vi "ControlPanel(noobjects.vi"() -> ()   [LabVIEW 2017]
panel:
  out "boot up output":string="\r\n"
  in  "Read":bool
  in  "Inhibit":bool
  in  "Change Wavelength in nm":bool
  in  "Change Retardance in nm":bool
  in  "Change Retardance in wave units":bool
  in  "Input":dbl
  out "Wavelength":dbl[unit]
  out "Retardation in nm":dbl[unit]
  out "Retardation in wave units":dbl
  in  "stop":bool
  out "error out":errorcluster
  in  "error in (no error)":errorcluster
  in  "Factory Reset":bool
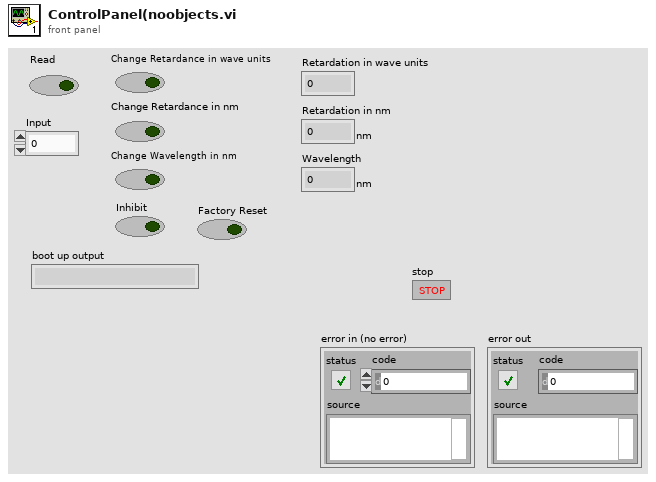
[diagram p1: front panel]
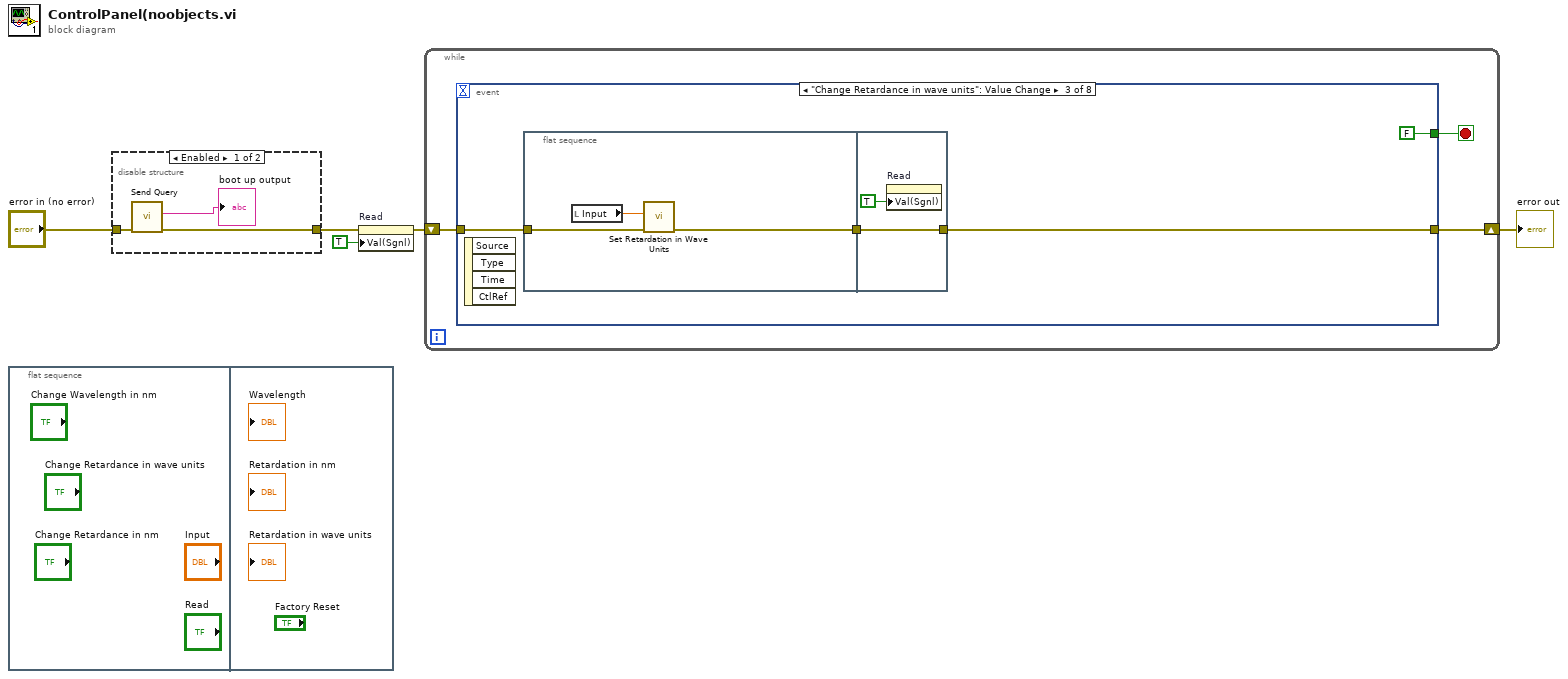
[diagram p0: block diagram]
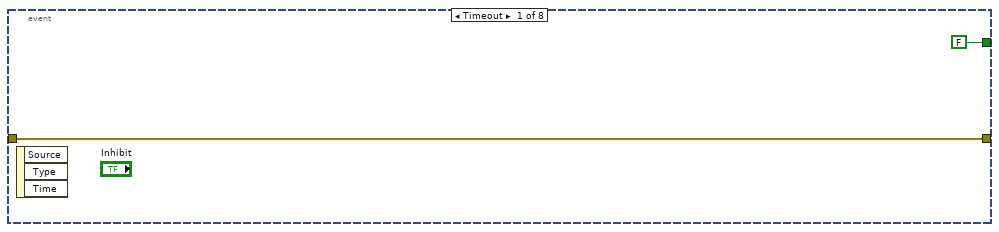
[diagram p3: hidden frame]
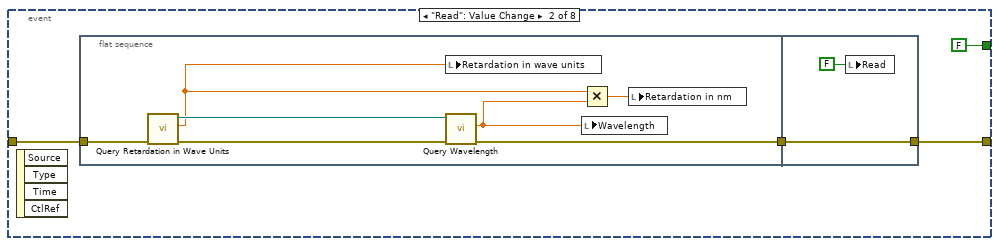
[diagram p4: hidden frame]
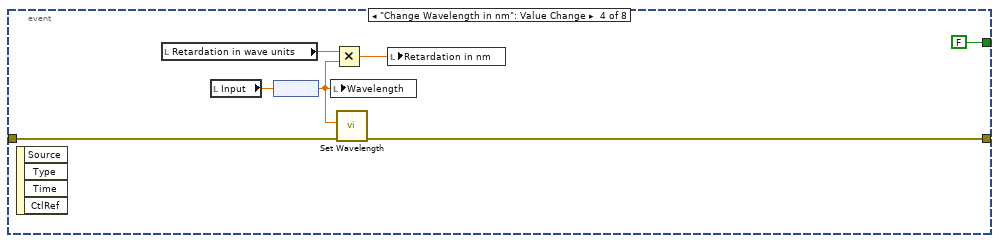
[diagram p5: hidden frame]
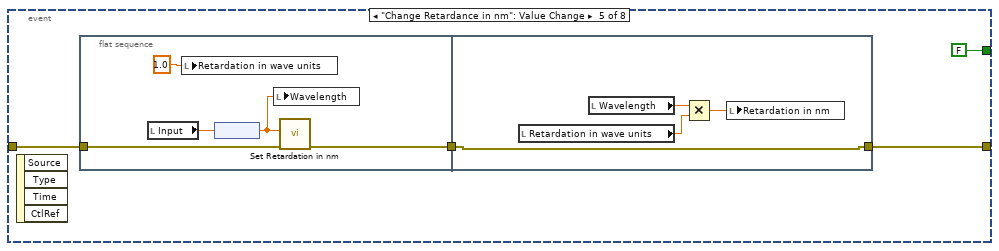
[diagram p6: hidden frame]
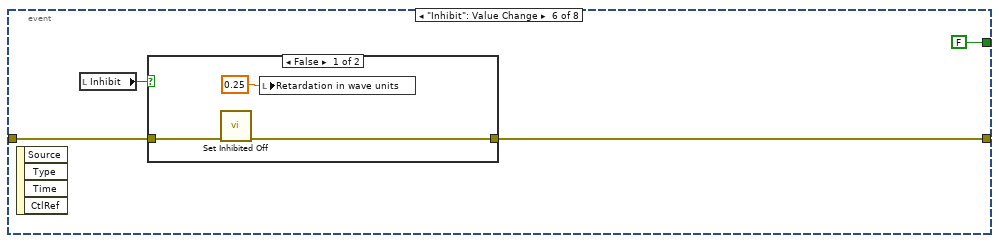
[diagram p7: hidden frame]
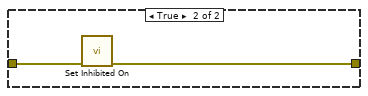
[diagram p8: hidden frame]
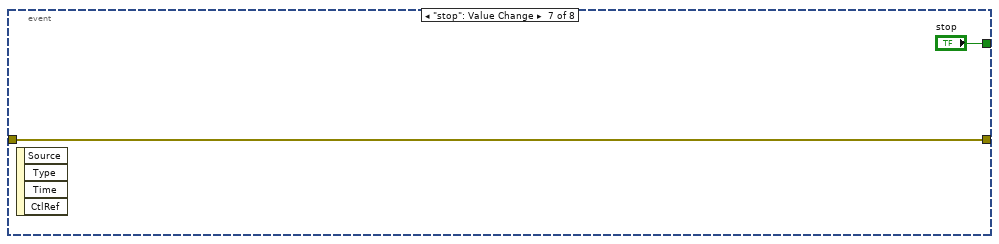
[diagram p9: hidden frame]
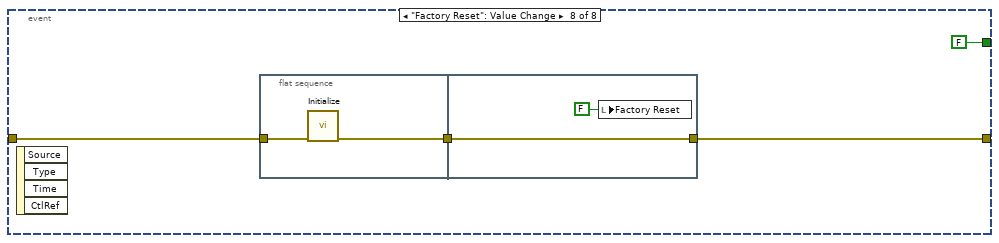
[diagram p10: hidden frame]
diagram:
  n1 = flat-sequence {
    frame #0 {
    }
    frame #1 {
    }
  }
  n2 = disable-structure shown="Enabled" {
    disable-tunnel: "error in (no error)" -> [w8 w9]
    disable-tunnel: [w7 w9] -> w1
    frame Enabled {
      n3 = call "Send Query.vi"("error in (no error)"=w8) -> ("error out"=w7:errorcluster, "query output"=→"boot up output":string)  [unwired: 8 in, 1 out]
    }
    frame Disabled {
    }
  }
  n4 = property on="Read" class="Bool (strict)"(error in=w1, "Val(Sgnl)"=TRUE ("Value (Signaling)")) -> (error out=w4:errorcluster)  [unwired: 1 in, 1 out]
  n5 = while {
    shift-right: [w11] -> w5
    shift-left: w4 -> [w12]
    stop <- w10 stop-if-true
    n6 = event shown="[2] \"Change Retardance in wave units\": Value Change" {
      selector: _ -> [_ _ _ _ _ _ _ _]
      dyn-events: _ -> [_ _ _ _ _ _ _ _]
      timeout: _ -> [_ _ _ _ _ _ _ _]
      tunnel: w12 -> [w14 w17 w31 w42 w47 w58 w66 w71]
      tunnel: [w14 w16 w30 w41 w46 w57 w66 w70] -> w11
      tunnel: [FALSE ("Boolean") FALSE ("Boolean") FALSE ("Boolean") FALSE ("Boolean") FALSE ("Boolean") FALSE ("Boolean") "stop" FALSE ("Boolean")] -> w10
      event Timeout {
        n7 = event-data() -> ()  [unwired: 1 in, 3 out]
      }
      event "Read": Value Change {
        n8 = event-data() -> ()  [unwired: 1 in, 4 out]
        n9 = flat-sequence {
          tunnel: w17 -> [w25]
          tunnel: [w23] -> w15
          tunnel: [w27] -> w16
          tunnel: w15 -> [w27]
          frame #0 {
            n10 = call "Query Retardation in Wave Units.vi"("error in (no error)"=w25) -> ("error out"=w24:errorcluster, "Fraction of wave Retardation"=w20:dbl, "VISA resource name out"=w22:refnum<visa-resource-name>)  [unwired: 8 in]
            n11 = local write "Retardation in wave units"(w20) -> ()
            n12 = call "Query Wavelength.vi"("error in (no error)"=w24, "VISA resource name"=w22) -> ("error out"=w23:errorcluster, "Wavelength"=w19:dbl[unit])  [unwired: 7 in, 1 out]
            n13 = Multiply(x=w20, y=w19) -> (x*y=w21:dbl[unit])
            n14 = local write "Wavelength"(w19) -> ()
            n15 = local write "Retardation in nm"(w21) -> ()
          }
          frame #1 {
            n16 = local write "Read"(FALSE ("Read")) -> ()
          }
        }
      }
      event "Change Retardance in wave units": Value Change {
        n17 = event-data() -> ()  [unwired: 1 in, 4 out]
        n18 = flat-sequence {
          tunnel: w31 -> [w34]
          tunnel: [w33] -> w28
          tunnel: [w36] -> w30
          tunnel: w28 -> [w36]
          frame #0 {
            n19 = local read "Input"() -> (w32:dbl)
            n20 = call "Set Retardation in Wave Units.vi"("fraction of wave"=w32, "error in (no error)"=w34) -> ("error out"=w33:errorcluster)  [unwired: 7 in, 1 out]
          }
          frame #1 {
            n21 = property on="Read" class="Bool (strict)"("Val(Sgnl)"=TRUE ("Value (Signaling)")) -> ()  [unwired: 2 in, 2 out]
          }
        }
      }
      event "Change Wavelength in nm": Value Change {
        n22 = event-data() -> ()  [unwired: 1 in, 4 out]
        n23 = local read "Retardation in wave units"() -> (w37:dbl)
        n24 = local read "Input"() -> (w43:dbl)
        n25 = node(w43) -> (w38:dbl[unit])
        n26 = local write "Wavelength"(w38) -> ()
        n27 = Multiply(x=w37, y=w38) -> (x*y=w39:dbl[unit])
        n28 = call "Set Wavelength.vi"("error in (no error)"=w42, "wavelength"=w38) -> ("error out"=w41:errorcluster)  [unwired: 8 in, 1 out]
        n29 = local write "Retardation in nm"(w39) -> ()
      }
      event "Change Retardance in nm": Value Change {
        n30 = event-data() -> ()  [unwired: 1 in, 4 out]
        n31 = flat-sequence {
          tunnel: w47 -> [w52]
          tunnel: [w51] -> w44
          tunnel: [w56] -> w46
          tunnel: w44 -> [w56]
          frame #0 {
            n32 = local read "Input"() -> (w50:dbl)
            n33 = local write "Retardation in wave units"(1.0 ("Retardation in wave units")) -> ()
            n34 = node(w50) -> (w48:dbl[unit])
            n35 = local write "Wavelength"(w48) -> ()
            n36 = call "Set Retardation in nm.vi"("error in (no error)"=w52, "Retardance in nm"=w48) -> ("error out"=w51:errorcluster)  [unwired: 8 in, 1 out]
          }
          frame #1 {
            n37 = local read "Retardation in wave units"() -> (w54:dbl)
            n38 = local read "Wavelength"() -> (w55:dbl[unit])
            n39 = Multiply(x=w55, y=w54) -> (x*y=w53:dbl[unit])
            n40 = local write "Retardation in nm"(w53) -> ()
          }
        }
      }
      event "Inhibit": Value Change {
        n41 = event-data() -> ()  [unwired: 1 in, 4 out]
        n42 = local read "Inhibit"() -> (w60:bool)
        n43 = case shown="False" w60 {
          tunnel: w58 -> [w63 w65]
          tunnel: [w62 w64] -> w57
          frame False {
            n44 = call "Set Inhibited Off.vi"("error in (no error)"=w63) -> ("error out"=w62:errorcluster)  [unwired: 9 in, 1 out]
            n45 = local write "Retardation in wave units"(0.25 ("Retardation in wave units")) -> ()
          }
          frame True {
            n46 = call "Set Inhibited On.vi"("error in (no error)"=w65) -> ("error out"=w64:errorcluster)  [unwired: 9 in, 1 out]
          }
        }
      }
      event "stop": Value Change {
        n47 = event-data() -> ()  [unwired: 1 in, 4 out]
      }
      event "Factory Reset": Value Change {
        n48 = event-data() -> ()  [unwired: 1 in, 4 out]
        n49 = flat-sequence {
          tunnel: w71 -> [w73]
          tunnel: [w72] -> w68
          tunnel: [w75] -> w70
          tunnel: w68 -> [w75]
          frame #0 {
            n50 = call "Initialize.vi"("error in (no error)"=w73) -> ("error out"=w72:errorcluster)  [unwired: 8 in, 2 out]
          }
          frame #1 {
            n51 = local write "Factory Reset"(FALSE ("Factory Reset")) -> ()
          }
        }
      }
    }
  }
  "error out" <- w5
